vi "Create Sorted Profit List.vi"(11 "Stats since last update":T1[](array[typedef]) {"Date Updated" format="%<%m/%d/%Y>T"}) -> (2 "residual":dbl, 3 "Sorted by profit":cluster{"Player Name":string, "Profit":dbl}[](array[cluster]) {"Profit" format="%#.2g"})   [LabVIEW 2021]
uses:
  WPC Player and Financial Stats.ctl
  c5767470-97fa-49bb-9491-df30637d67ff.vi
  <vilib>/Array/Sort 2D Array - Pop Stack.vi
  <vilib>/Array/Sort 2D Array - Push Stack.vi
  c5767470-97fa-49bb-9491-df30637d67ff.vi/269d4b3b-47f5-49e3-8884-44851e4dd9d5.vi
  c5767470-97fa-49bb-9491-df30637d67ff.vi/6d99389c-673d-4efb-bf33-19b32bcf4cf8.vi
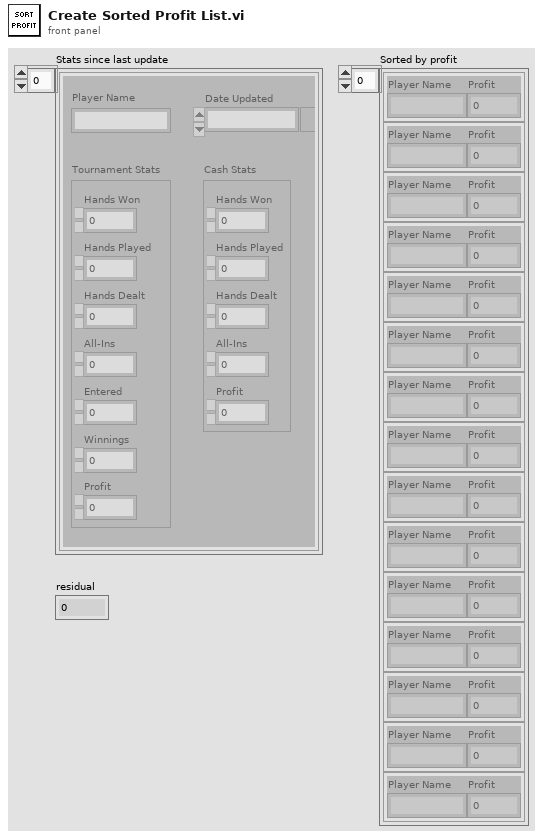
[diagram p1: front panel]
types:
  T1 = typedef "WPC Player and Financial Stats.ctl" = cluster{"Player Name":string, "Date Updated":timestamp, "Tournament Stats":cluster{"Hands Won":i32, "Hands Played":i32, "Hands Dealt":i32, "All-Ins":i32, "Entered":i32, "Winnings":dbl, "Profit":dbl}, "Cash Stats":cluster{"Hands Won":i32, "Hands Played":i32, "Hands Dealt":i32, "All-Ins":i32, "Profit":dbl}}
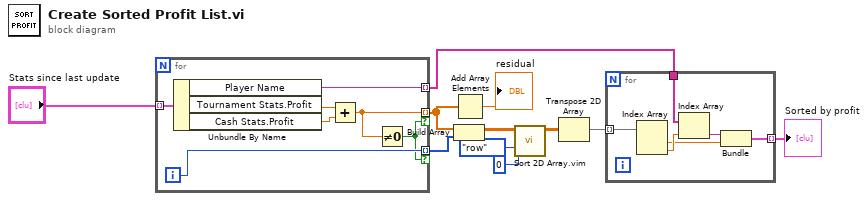
[diagram p0: block diagram]
diagram:
  n1 = for {
    tunnel: "Stats since last update" -> [w18] mode=indexing
    tunnel: [w17] -> w4 mode=indexing
    tunnel: [w14] -> w2 mode=indexing if=w12
    tunnel: [w13] -> w10 mode=indexing if=w12
    i -> [w13]
    n2 = Unbundle By Name(w18) -> ("Player Name"=w17:string, "Tournament Stats.Profit"=w16:dbl, "Cash Stats.Profit"=w15:dbl)
    n3 = Add(x=w16, y=w15) -> (x+y=w14:dbl)
    n4 = Not Equal To 0?(x=w14) -> (x != 0?=w12:bool)
  }
  n5 = Build Array(w2, w10) -> (w9:dbl[][])
  n6 = Add Array Elements(numeric array=w2) -> (sum=→"residual":dbl)
  n7 = call "Sort 2D Array.vim"("index"=0, "dimension to index (column)"=enum16{"column", "row"}."row", "2D array"=w9) -> ("sorted 2D array"=w6:dbl[][])  [unwired: 7 in, 1 out]
  n8 = Transpose 2D Array(2D array=w6) -> (transposed array=w5:dbl[][])
  n9 = for {
    tunnel: w5 -> [w24] mode=indexing
    tunnel: w4 -> [w23]
    tunnel: [w19] -> w3 mode=indexing
    n10 = Index Array(array=w24) -> (element #1=w20:dbl, element #2=w22:dbl)  [unwired: 2 in]
    n11 = Index Array(array=w23, index=w22) -> (element=w21:string)
    n12 = Bundle("Player Name"=w21, w20) -> (w19:cluster{"Player Name":string, dbl})  [unwired: 1 in]
  }
  "Sorted by profit" <- w3
